vi "PWM Modified 3 (FPGA).vi"(2 "PWM Period (Ticks)":u32=40000, 3 "PWM Duty Cycle (Ticks)":i32, 6 "Min Period (Ticks)":u32=1000) -> (15 "PWM DO":bool, 16 "PWM Clock":bool, 17 "Changed?":bool, 18 "Telapsed (Ticks)":u32)   [LabVIEW 2019]
doc: "Generates a digital pulse width modulation (PWM) signal. PWM signals are useful for driving loads such as motors and proportional valves because the average voltage supplied is equal to the PWM duty cycle. The output of this function can be connected to digital output modules. This function is designed for use in LabVIEW FPGA.\n\nOPERATION\nAt the beginning of each cycle the digital output is turned on. The digital output is left on for the amount of time specified by the PWM Duty Cycle (Ticks) input. The cycle repeats when the amount of time specified by the PWM Period (Ticks) has elapsed. The FPGA tick counter is used to calculate elapsed time. By default, one tick is equal to 25 nanoseconds (40 MHz), so a PWM Period (Ticks) of 40,000 results in a 1 kHz PWM signal. The PWM Duty Cycle (Ticks) input is a signed integer, but the sign of the value is ignored.\n\nThis subVI is reentrant, so you can place multiple instances of the function in a LabVIEW FPGA application and they each will operate independently.\n\nTo obtain the highest timing resolution when using this function in a loop, you can perform digital output I/O operations only when the PWM DO value has changed (rather than on every cycle). To do this, wire the Changed? output to the conditional terminal on a case statement and perform the I/O operation when the case statement is True. If the duty cycle is 0 or 100%, the Changed? output will strobe true once per PWM cycle at the beginning of the cycle.\n\nThe PWM Clock signal is a 50% duty cycle square wave signal that can be used to synchronize other loops with the beginning (rising edge) or middle (falling edge) of the PWM cycle.\n\nThe Telapsed (Ticks) signal can be used to trigger other operations at particular time in the PWM cycle. For instance, you could use this signal to trigger an analog input operation to occur once per PWM cycle at a programmable time within the PWM cycle. This counter resets back to 0 at the beginning of every PWM cycle.\n\nThe Min Period (Ticks) signal is used to limit the PWM Period to prevent switching at frequencies that could damage the output MOSFETs in a digital output device. By default Min Period (Ticks) is set to 1000 ticks, which limits the PWM switching frequency to 40 kHz.\n\nINPUTS\nPWM Period (Ticks)- Total width of the pulse (inverse of the \"PWM Frequency\")\nPWM Duty Cycle (Ticks)- Time for which signal output stays True\nMin Period (Ticks)- The minimum allowed value for the PWM Period \n\nOUTPUTS\nPWM DO- Digital PWM signal that can be connected to a digital output channel I/O node\nPWM Clock- 50% duty cycle clock signal that can be used for synchronizing other loops\nChanged?- Value is True for one iteration when the PWM DO value has changed, or at the beginning of the PWM cycle if the duty cycle is 0 or 100%\nTelapsed- The amount of time elapsed during the current PWM cycle\n\nSCALING\n\nThe formulas below can be used for scaling from units of Hz, seconds, or percent duty cycle in the real-time host interface application. These formulas assume a 40 MHz (40,000,000 Ticks/sec) FPGA clock rate.\n\nPWM Period (Ticks) = 40,000,000 / PWM Period (Hz)\nPWM Period (Ticks) = 40,000,000 * PWM Period (sec)\nPWM Duty Cycle (Ticks) = PWM Period (Ticks) * PWM Duty Cycle (%) / 100\nPWM Duty Cycle (Ticks) = 40,000,000 * PWM Duty Cycle (sec)"
uses:
  <vilib>/Platform/TimedLoop/XDataNode/timing_clust.ctl
  <vilib>/Platform/TimedLoop/XDataNode/nitl_modes.ctl
  <vilib>/Platform/TimedLoop/XDataNode/wakeup.ctl
  <vilib>/rvi/Emulation/niFpgaSctlEmulationGetInTimedLoop.vi
  <vilib>/rvi/Emulation/niFpgaEmulationReportErrorSimple.vi
  <vilib>/rvi/Emulation/niFpgaGetClockAttributes.vi
  <vilib>/rvi/Emulation/niFpgaCriticalErrorInLSC.vi
  Instance           5 37Saved   Pulse Width Modulation (FPGA) .vi
  Instance           6 37Saved   Pulse Width Modulation (FPGA) .vi
  <vilib>/Platform/TimedLoop/XDataNode/XDataNode.xnode
  <vilib>/Platform/TimedLoop/XDataNode/XDNodeRunTimeDep.lvlib
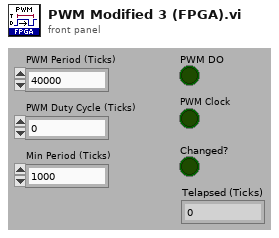
[diagram p1: front panel]
types:
  T1 = typedef "XDNodeRunTimeDep.lvlib/timing_clust.ctl" = cluster{"Expected End [f-1]":u64, "Actual End [f-1]":u64, "Finished Late? [f-1]":bool, "Expected End [i-1]":u64, "Actual End [i-1]":u64, "Finished Late? [i-1]":bool, "Expected Start [i]":u64, "Actual Start [i]":u64, "Expected Start [f]":u64, "Actual Start [f]":u64, "Source Name":string, "Structure Name":string, "Period":i64, "Deadline":i64, "Offset":i64, "Start":i64, "Priority":i32, "Timeout":i32, "Mode":T2, "Wakeup Reason":T3, "Error":errorcluster, "Source Type":string, "Secondary Source Type":string, "Global End Time":u64, "Global Start Time":u64, "Frame Duration":u64, "Iteration Duration":u64, "Assigned CPU":i32, "I/O Scan Engine Mode":u32}
  T2 = typedef "XDNodeRunTimeDep.lvlib/nitl_modes.ctl" = enum32{"No Change", "Process missed periods, maintain original phase", "Discard missed periods, maintain original phase", "Process missed periods, ignore original phase", "Discard missed periods, ignore original phase"}
  T3 = typedef "XDNodeRunTimeDep.lvlib/wakeup.ctl" = enum32{"Normal", "Aborted", "Asynchronous wakeup", "Timing source error", "Timed loop error", "Timeout"}
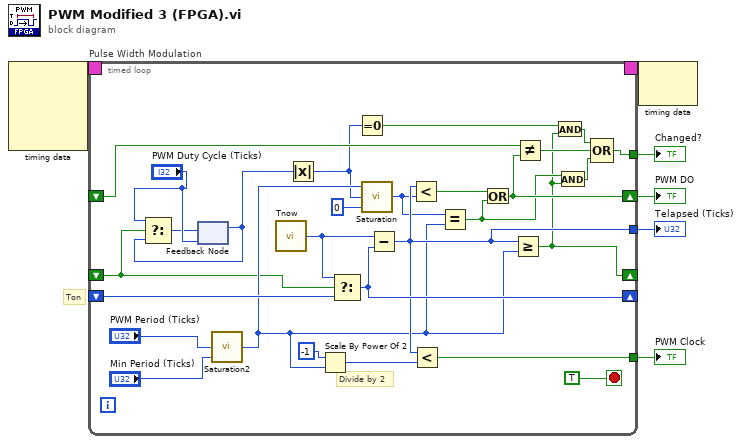
[diagram p0: block diagram]
diagram:
  # "Ton"
  n1 = node-c288() -> (w2:T1)  [unwired: 4 in]
  n2 = timed-loop "Pulse Width Modulation" {
    shift-right: [w31] -> _
    shift-left: _ -> [w32]
    shift-right: [w13] -> _
    shift-left: _ -> [w10]
    tunnel: [w28] -> w6
    tunnel: [w27] -> w5
    shift-right: [w16] -> w4
    shift-left: _ -> [w26]
    tunnel: [w18] -> w3
    timing: w2 -> [_]
    timing-out: [_] -> w1
    stop <- TRUE stop-if-true
    # "Divide by 2"
    n3 = feedback #1("PWM Duty Cycle (Ticks)") -> (w7:i32)
    n4 = Select(t="PWM Duty Cycle (Ticks)", s=w10, f=w7) -> (s? t:f=w8:i32)
    n5 = feedback-in #1(w8) -> ()
    n6 = call "Saturation2"("input"="PWM Period (Ticks)", "lower limit"="Min Period (Ticks)") -> ("output"=w22:u32)  [unwired: 7 in]
    n7 = call "Tnow"() -> ("Tick Count(Ticks)"=w33:u32)
    n8 = Absolute Value(x=w7) -> (abs(x)=w12:i32)
    n9 = Scale By Power Of 2(n=i8 -1, x=w22) -> (x*2^n=w30:u32)
    n10 = Select(t=w33, s=w10, f=w32) -> (s? t:f=w31:u32)
    n11 = Equal To 0?(x=w12) -> (x = 0?=w11:bool)
    n12 = call "Saturation"("upper limit"=w22, "input"=w12, "lower limit"=u32 0) -> ("output"=w23:u32)  [unwired: 6 in]
    n13 = Subtract(x=w33, y=w31) -> (x-y=w28:u32)
    n14 = Less?(x=w28, y=w23) -> (x < y?=w21:bool)
    n15 = Less?(x=w28, y=w30) -> (x < y?=w27:bool)
    n16 = Equal?(x=w23, y=w22) -> (x = y?=w15:bool)
    n17 = Or(x=w21, y=w15) -> (x .or. y?=w16:bool)
    n18 = Greater Or Equal?(x=w28, y=w22) -> (x >= y?=w13:bool)
    n19 = Not Equal?(x=w26, y=w16) -> (x != y?=w25:bool)
    n20 = And(x=w11, y=w13) -> (x .and. y?=w14:bool)
    n21 = And(x=w15, y=w13) -> (x .and. y?=w17:bool)
    n22 = Compound Arithmetic op=OR(w14, w25, w17) -> (w18:bool)
  }
  "Telapsed (Ticks)" <- w6
  "PWM Clock" <- w5
  "PWM DO" <- w4
  "Changed?" <- w3
  n23 = node-c288(w1) -> ()  [unwired: 1 out]
